vi "Create Antinodes Harmonics.vi"(7 "Max Grid Index":T1, 10 "Antena 2":T1, 11 "Antena 1":T1) -> (3 "Antinodes":T1[](array[typedef]))   [LabVIEW 2024]
uses:
  Cluster_Position.ctl
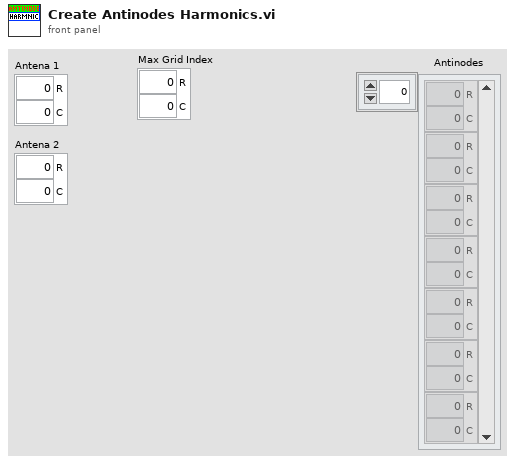
[diagram p1: front panel]
types:
  T1 = typedef "Cluster_Position.ctl" = cluster{"R":i32, "C":i32}
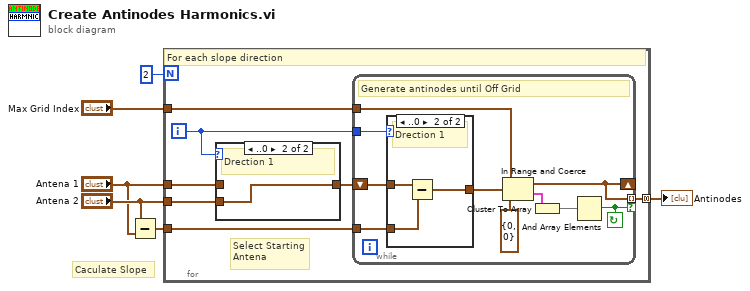
[diagram p0: block diagram]
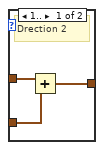
[diagram p3: hidden frame]
diagram:
  # "Caculate Slope"
  n1 = Subtract(x="Antena 2", y="Antena 1") -> (x-y=w2:T1)
  n2 = for {
    N: 2 -> [_]
    tunnel: w2 -> [w13]
    tunnel: "Antena 1" -> [w12]
    tunnel: "Antena 2" -> [w8]
    tunnel: "Max Grid Index" -> [w11]
    tunnel: [w7] -> w6 mode=concatenating
    i -> [w9]
    # "Select Starting\nAntena"
    # "For each slope direction"
    n3 = case shown="..0" w9 {
      tunnel: w12 -> [w14 _]
      tunnel: [w14 w15] -> w10
      tunnel: w8 -> [_ w15]
      frame 1.. {
        # "Drection 2"
      }
      frame ..0 {
        # "Drection 1"
      }
    }
    n4 = while {
      tunnel: w13 -> [w23]
      shift-right: [w20] -> _
      shift-left: w10 -> [w24]
      tunnel: w11 -> [w21]
      tunnel: w9 -> [w25]
      tunnel: [w20] -> w7 mode=indexing if=w16
      stop <- w16 continue-if-true
      # "Generate antinodes until Off Grid"
      n5 = case shown="..0" w25 {
        tunnel: w24 -> [w28 w31]
        tunnel: w23 -> [w27 w30]
        tunnel: [w26 w29] -> w22
        frame 1.. {
          # "Drection 2"
          n6 = Add(x=w28, y=w27) -> (x+y=w26:T1)
        }
        frame ..0 {
          # "Drection 1"
          n7 = Subtract(x=w31, y=w30) -> (x-y=w29:T1)
        }
      }
      n8 = In Range and Coerce(upper limit=w21, x=w22, lower limit=T1 {"R"=0, "C"=0}) -> (coerced(x)=w20:T1, In Range?=w18:cluster{"R":bool, "C":bool})
      n9 = Cluster To Array(cluster=w18) -> (array=w17:bool[])
      n10 = And Array Elements(Boolean array=w17) -> (logical AND=w16:bool)
    }
  }
  "Antinodes" <- w6
